vi "main_loop_calculation.vi"(0 "DAQ Data":waveform(dbl)[](array[waveform]), 1 "Offset Parameters":T1={"Separator \nTemperature"=0.0, "Separator Pressure"=0.0, "Lower Test Section\nTemperature"=0.0, "Lower Test Section\nPressure"=0.0, "Vapor Tank (Top) \nHeater"=0.0, "Liquid Tank (Bottom) \nHeater"=0.0, "Vapor Tank\nTemperature Offset"=0.0, "Vapor Tank\nPressure "=0.0, "Upper Test Section\nTemperature"=0.0, "Upper Test Section\nPressure"=0.0, "Vapor Inlet \nTemperature"=0.0, "Dev Section\nPressure"=0.0, "Liquid Tank\nTemperature"=0.0, "Liquid Tank\nPressure"=0.0, "Liquid Inlet\nTemperature "=0.0, "Liquid Inlet\nPressure"=0.0, "Atmospheric Pressure [Pa]"=101325.0}) -> (2 "Vapor Flow Data":T3, 3 "Liquid Flow Data":T2, 4 "Pressure/Temperature/Mixture Properties":T4)   [LabVIEW 2015]
panel:
  out "dt":dbl
  out "t0":timestamp
  out "Separator Temp. [C]":dbl
  out "Liquid Inlet T":dbl
  out "Vapor Inlet T Sat":dbl
  # "Saturation\nPressure [Pa]"
  # "Saturation\nTemperature [C]"
  # "Pressure [Pa]"
  # "Temperature [C]"
  # "Lower Test Section"
  # "Upper Test Section"
  # "Vapor Inlet\n(Dev Section)"
  # "Vapor Tank"
  # "Liquid Inlet"
  # "Separator"
  # "Liquid Tank"
  # "Streamwise(dP)"
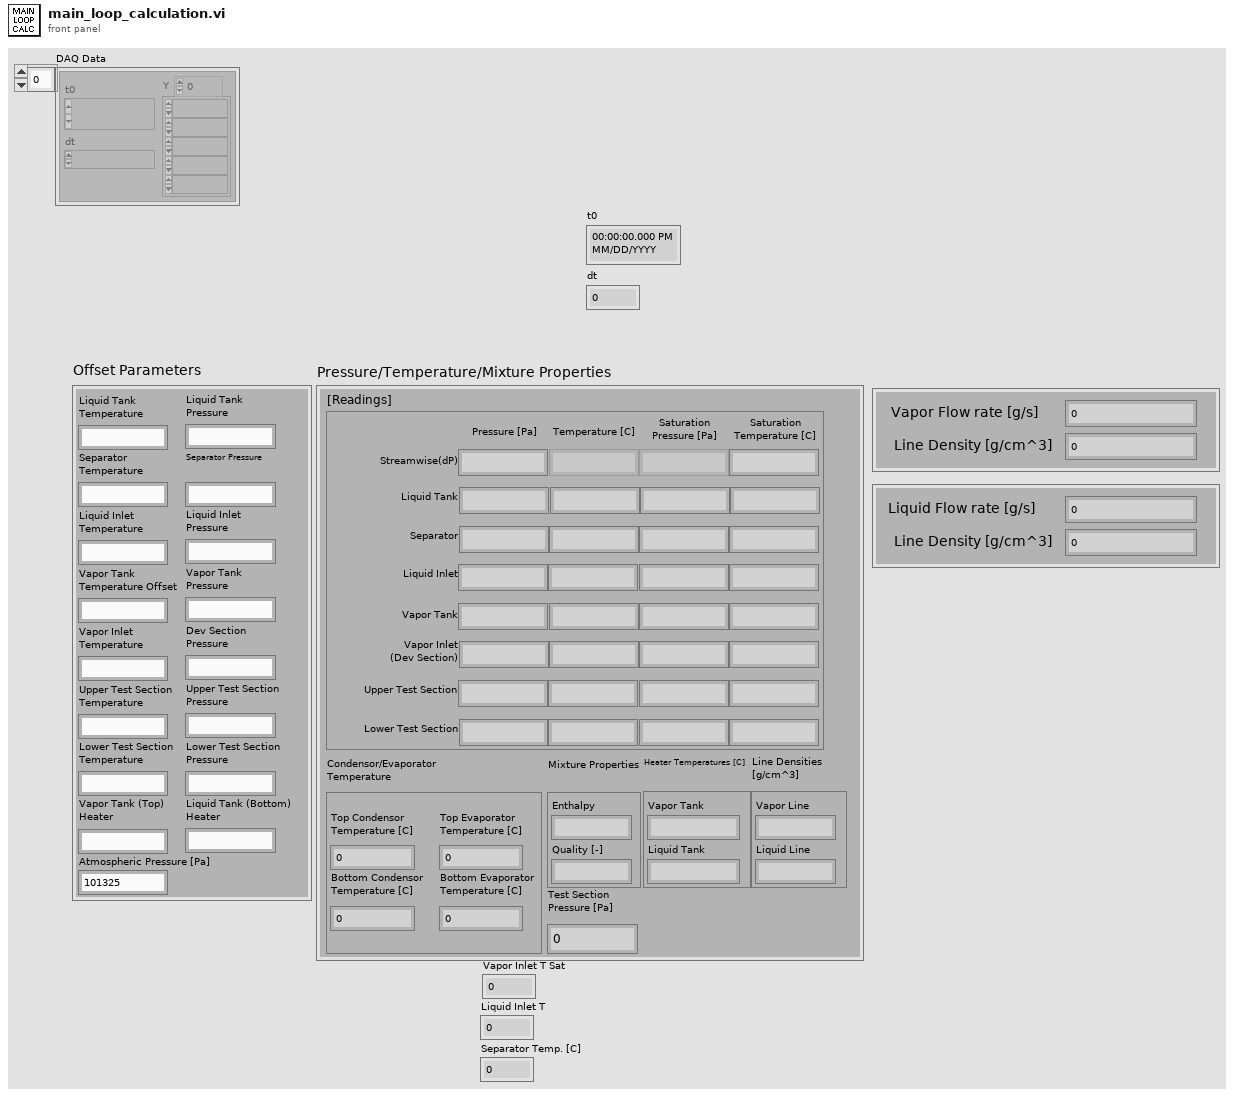
[diagram p1: front panel]
types:
  T1 = cluster{"Separator \nTemperature":dbl, "Separator Pressure":dbl, "Lower Test Section\nTemperature":dbl, "Lower Test Section\nPressure":dbl, "Vapor Tank (Top) \nHeater":dbl, "Liquid Tank (Bottom) \nHeater":dbl, "Vapor Tank\nTemperature Offset":dbl, "Vapor Tank\nPressure ":dbl, "Upper Test Section\nTemperature":dbl, "Upper Test Section\nPressure":dbl, "Vapor Inlet \nTemperature":dbl, "Dev Section\nPressure":dbl, "Liquid Tank\nTemperature":dbl, "Liquid Tank\nPressure":dbl, "Liquid Inlet\nTemperature ":dbl, "Liquid Inlet\nPressure":dbl, "Atmospheric Pressure [Pa]":dbl}
  T2 = cluster{"Liquid Flow rate [g/s]":dbl, "Line Density [g/cm^3]":dbl}
  T3 = cluster{"Vapor Flow rate [g/s]":dbl, "Line Density [g/cm^3]":dbl}
  T4 = cluster{"Line Densities\n[g/cm^3]":cluster{"Vapor Line":dbl, "Liquid Line":dbl}, "Mixture Properties":cluster{"Enthalpy":dbl, "Quality [-]":dbl}, "[Readings]":cluster{"Streamwise P":dbl, "Streamwise T":dbl, "Streamwise Sat P":dbl, "Streamwise Sat T":dbl, "Liquid Tank P":dbl, "Liquid Tank T":dbl, "Liquid Tank Sat P":dbl, "Liquid Tank Sat T":dbl, "Separator P":dbl, "Separator T":dbl, "Separator Sat P":dbl, "Separator Sat T":dbl, "Liquid Inlet P":dbl, "Liquid Inlet T":dbl, "Liquid Inlet Sat P":dbl, "Liquid Inlet Sat T":dbl, "Vapor Tank P":dbl, "Vapor Tank T":dbl, "Vapor Tank Sat P":dbl, "Vapor Tank Sat T":dbl, "Vapor Inlet P":dbl, "Vapor Inlet T":dbl, "Vapor Inlet Sat P":dbl, "Vapor Inlet Sat T":dbl, "Upper Test Section P":dbl, "Upper Test Section T":dbl, "Upper Test Section Sat P":dbl, "Upper Test Section Sat T":dbl, "Lower Test Section P":dbl, "Lower Test Section T":dbl, "Lower Test Section Sat P":dbl, "Lower Test Section Sat T":dbl}, "Condensor/Evaporator\nTemperature":cluster{"Bottom Evaporator\nTemperature [C]":dbl, "Bottom Condensor\nTemperature [C]":dbl, "Top Evaporator\nTemperature [C]":dbl, "Top Condensor\nTemperature [C]":dbl}, "Test Section \nPressure [Pa]":dbl, "Heater Temperatures [C]":cluster{"Vapor Tank":dbl, "Liquid Tank":dbl}}
  T5 = cluster{"[0]":dbl, "[1]":dbl, "[2]":dbl, "[3]":dbl}
  T6 = cluster{"mixture enthalpy":dbl, "Quality [-]":dbl}
  T7 = cluster{"array[0]":dbl, "array[1]":dbl, "array[2]":dbl, "array[3]":dbl, "array[4]":dbl, "array[5]":dbl, "array[6]":dbl, "array[7]":dbl, "array[8]":dbl, "array[9]":dbl, "array[10]":dbl, "array[11]":dbl, "array[12]":dbl, "array[13]":dbl, "array[14]":dbl, "array[15]":dbl, "array[16]":dbl, "array[17]":dbl, "array[18]":dbl, "array[19]":dbl, "array[20]":dbl, "array[21]":dbl, "array[22]":dbl, "array[23]":dbl, "array[24]":dbl, "array[25]":dbl, "array[26]":dbl, "array[27]":dbl, "array[28]":dbl, "array[29]":dbl, "array[30]":dbl, "array[31]":dbl}
  T8 = cluster{cluster{"[0]":dbl, "[1]":dbl}, cluster{"mixture enthalpy":dbl, "Quality [-]":dbl}, "Cluster":cluster{"array[0]":dbl, "array[1]":dbl, "array[2]":dbl, "array[3]":dbl, "array[4]":dbl, "array[5]":dbl, "array[6]":dbl, "array[7]":dbl, "array[8]":dbl, "array[9]":dbl, "array[10]":dbl, "array[11]":dbl, "array[12]":dbl, "array[13]":dbl, "array[14]":dbl, "array[15]":dbl, "array[16]":dbl, "array[17]":dbl, "array[18]":dbl, "array[19]":dbl, "array[20]":dbl, "array[21]":dbl, "array[22]":dbl, "array[23]":dbl, "array[24]":dbl, "array[25]":dbl, "array[26]":dbl, "array[27]":dbl, "array[28]":dbl, "array[29]":dbl, "array[30]":dbl, "array[31]":dbl}, cluster{"[0]":dbl, "[1]":dbl, "[2]":dbl, "[3]":dbl}, "Absolute Pressure [Pa]":dbl, cluster{"[0]":dbl, "[1]":dbl}}
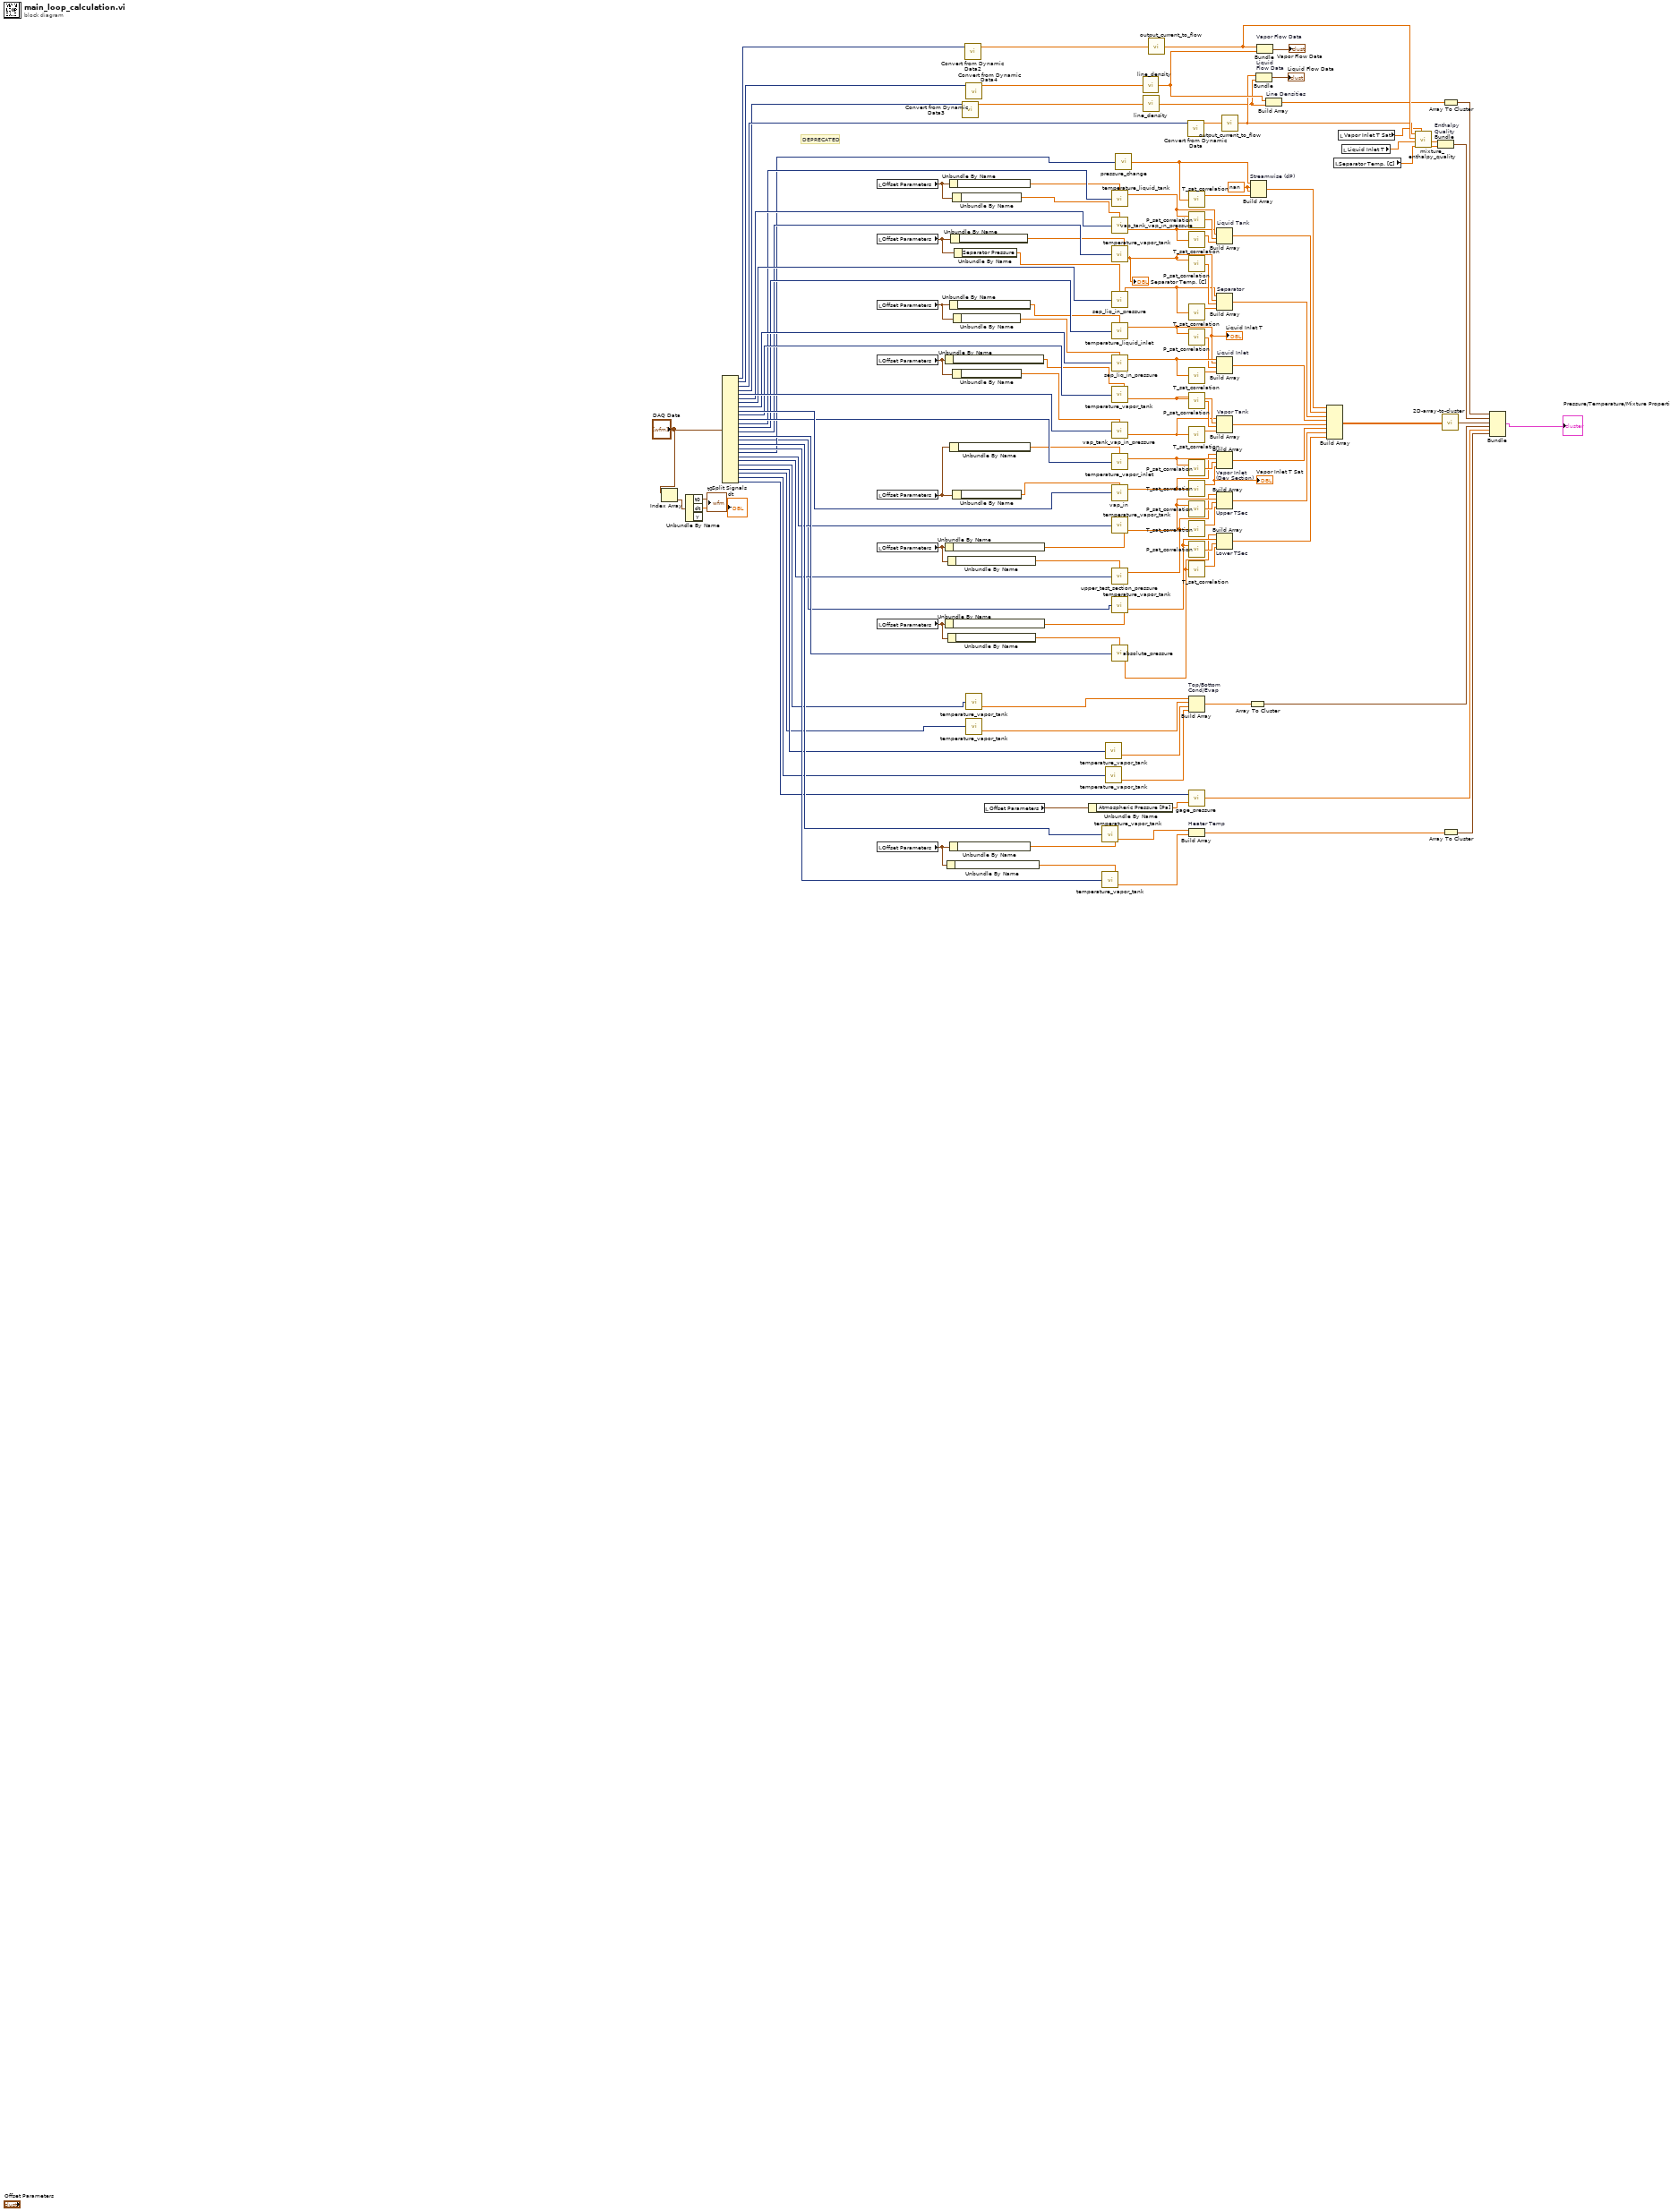
[diagram p0: block diagram]
diagram:
  w93 = nan
  # "DEPRECATED"
  n1 = Index Array(array="DAQ Data") -> (element=w3:waveform(dbl))  [unwired: 1 in]
  n2 = Unbundle By Name(w3) -> ("t0"=→"t0":timestamp, "dt"=→"dt":dbl)  [unwired: 1 out]
  n3 = Split Signals("DAQ Data") -> (w38:dynamicdata, w21:dynamicdata, w126:dynamicdata, w125:dynamicdata, w124:dynamicdata, w123:dynamicdata, w122:dynamicdata, w121:dynamicdata, w120:dynamicdata, w119:dynamicdata, w118:dynamicdata, w117:dynamicdata, w116:dynamicdata, w115:dynamicdata, w114:dynamicdata, w20:dynamicdata, w113:dynamicdata, w112:dynamicdata, w74:dynamicdata, w111:dynamicdata, w110:dynamicdata, w18:dynamicdata, w109:dynamicdata, w17:dynamicdata, w105:dynamicdata, w103:dynamicdata)  [unwired: 26 in]
  n4 = local read "Offset Parameters"() -> (w56:T1)
  n5 = local read "Offset Parameters"() -> (w52:T1)
  n6 = local read "Offset Parameters"() -> (w51:T1)
  n7 = local read "Offset Parameters"() -> (w58:T1)
  n8 = local read "Offset Parameters"() -> (w53:T1)
  n9 = local read "Offset Parameters"() -> (w54:T1)
  n10 = local read "Offset Parameters"() -> (w55:T1)
  n11 = local read "Offset Parameters"() -> (w57:T1)
  n12 = Unbundle By Name(w54) -> ("Upper Test Section\nTemperature"=w66:dbl)
  n13 = Unbundle By Name(w55) -> ("Lower Test Section\nTemperature"=w19:dbl)
  n14 = Unbundle By Name(w58) -> ("Vapor Tank\nTemperature Offset"=w68:dbl)
  n15 = Unbundle By Name(w57) -> ("Liquid Tank (Bottom) \nHeater"=w69:dbl)
  n16 = Unbundle By Name(w54) -> ("Upper Test Section\nPressure"=w65:dbl)
  n17 = Unbundle By Name(w55) -> ("Lower Test Section\nPressure"=w71:dbl)
  n18 = Unbundle By Name(w56) -> ("Liquid Tank\nTemperature"=w62:dbl)
  n19 = Unbundle By Name(w51) -> ("Liquid Inlet\nTemperature"=w60:dbl)
  n20 = Unbundle By Name(w57) -> ("Vapor Tank (Top) \nHeater"=w70:dbl)
  n21 = Unbundle By Name(w53) -> ("Vapor Inlet \nTemperature"=w64:dbl)
  n22 = Unbundle By Name(w52) -> ("Separator \nTemperature"=w73:dbl)
  n23 = Unbundle By Name(w56) -> ("Liquid Tank\nPressure"=w61:dbl)
  n24 = Unbundle By Name(w58) -> ("Vapor Tank\nPressure"=w67:dbl)
  n25 = Unbundle By Name(w53) -> ("Dev Section\nPressure"=w63:dbl)
  n26 = Unbundle By Name(w51) -> ("Liquid Inlet\nPressure"=w59:dbl)
  n27 = Unbundle By Name(w52) -> ("Separator Pressure"=w72:dbl)
  n28 = call "Convert from Dynamic Data3"("Dynamic Data Type"=w125) -> ("Array"=w23:dbl[])  [unwired: 3 in]
  n29 = call "Convert from Dynamic Data2"("Dynamic Data Type"=w38) -> ("Array"=w37:dbl[])  [unwired: 3 in]
  n30 = call "Convert from Dynamic Data4"("Dynamic Data Type"=w21) -> ("Array"=w22:dbl[])  [unwired: 3 in]
  n31 = call "temperature_vapor_tank.vi"("Temp. Voltage\n[V]"=w18) -> ("Offset Temp. [C]"=w108:dbl)  [unwired: 3 in]
  n32 = call "temperature_vapor_tank.vi"("Temp. Voltage\n[V]"=w17) -> ("Offset Temp. [C]"=w107:dbl)  [unwired: 3 in]
  n33 = local read "Offset Parameters"() -> (w42:T1)
  n34 = Unbundle By Name(w42) -> ("Atmospheric Pressure [Pa]"=w41:dbl)
  n35 = call "temperature_vapor_tank.vi"("Offset [C]"=w70, "Temp. Voltage\n[V]"=w113) -> ("Offset Temp. [C]"=w76:dbl)  [unwired: 2 in]
  n36 = call "temperature_vapor_tank.vi"("Offset [C]"=w69, "Temp. Voltage\n[V]"=w112) -> ("Offset Temp. [C]"=w75:dbl)  [unwired: 2 in]
  n37 = call "temperature_vapor_tank.vi"("Temp. Voltage\n[V]"=w109) -> ("Offset Temp. [C]"=w106:dbl)  [unwired: 3 in]
  n38 = call "temperature_vapor_tank.vi"("Temp. Voltage\n[V]"=w105) -> ("Offset Temp. [C]"=w104:dbl)  [unwired: 3 in]
  n39 = call "temperature_liquid_tank.vi"("Offset [C]"=w62, "Temp. Voltage\n[V]"=w117) -> ("Temp. [C]"=w102:dbl)  [unwired: 2 in, 1 out]
  n40 = call "vap_tank_vap_in_pressure.vi"("Offset [Pa]"=w61, "Abs. Pressure\nVoltage [V]"=w123) -> ("Offset Absolute Pressure [Pa]"=w88:dbl)  [unwired: 2 in, 1 out]
  n41 = call "temperature_vapor_tank.vi"("Offset [C]"=w73, "Temp. Voltage\n[V]"=w115) -> ("Offset Temp. [C]"=w35:dbl)  [unwired: 2 in]
  "Separator Temp. [C]" <- w35
  n42 = call "sep_liq_in_pressure.vi"("Offset [Pa]"=w72, "Abs. Pressure\nVoltage [V]"=w122) -> ("Absolute Pressure [Pa]"=w16:dbl)  [unwired: 2 in, 1 out]
  n43 = call "temperature_liquid_inlet.vi"("Offset [C]"=w60, "Temp. Voltage\n[V]"=w116) -> ("Temp. [C]"=w34:dbl)  [unwired: 2 in, 1 out]
  "Liquid Inlet T" <- w34
  n44 = call "sep_liq_in_pressure.vi"("Offset [Pa]"=w59, "Abs. Pressure\nVoltage [V]"=w121) -> ("Absolute Pressure [Pa]"=w85:dbl)  [unwired: 2 in, 1 out]
  n45 = call "temperature_vapor_tank.vi"("Offset [C]"=w68, "Temp. Voltage\n[V]"=w119) -> ("Offset Temp. [C]"=w92:dbl)  [unwired: 2 in]
  n46 = call "vap_tank_vap_in_pressure.vi"("Offset [Pa]"=w67, "Abs. Pressure\nVoltage [V]"=w124) -> ("Offset Absolute Pressure [Pa]"=w87:dbl)  [unwired: 2 in, 1 out]
  n47 = call "temperature_vapor_inlet.vi"("Offset [C]"=w64, "Temp. Voltage\n[V]"=w118) -> ("Temp. [C]"=w95:dbl)  [unwired: 2 in, 1 out]
  n48 = call "vap_in.vi"("Offset [Pa]"=w63, "Abs. Pressure\nVoltage [V]"=w120) -> ("Absolute Pressure [Pa]"=w24:dbl)  [unwired: 2 in, 1 out]
  n49 = call "temperature_vapor_tank.vi"("Offset [C]"=w66, "Temp. Voltage\n[V]"=w111) -> ("Offset Temp. [C]"=w78:dbl)  [unwired: 2 in]
  n50 = call "upper_test_section_pressure.vi"("Offset [Pa]"=w65, "Waveform Graph"=w110) -> ("Absolute Pressure [Pa]"=w77:dbl)  [unwired: 2 in, 1 out]
  n51 = call "temperature_vapor_tank.vi"("Offset [C]"=w19, "Temp. Voltage\n[V]"=w20) -> ("Offset Temp. [C]"=w91:dbl)  [unwired: 2 in]
  n52 = call "absolute_pressure.vi"("Offset [V]"=w71, "Abs. Pressure\nVoltage [V]"=w114) -> ("Offset Absolute Pressure [Pa]"=w86:dbl)  [unwired: 2 in, 1 out]
  n53 = call "pressure_change.vi"("Pressure Voltage (V)"=w74) -> ("Streamwise dP (kPa)"=w99:dbl)
  n54 = call "line_density.vi"("DensCurr"=w22) -> ("Line Density"=w29:dbl)
  n55 = call "line_density.vi"("DensCurr"=w23) -> ("Line Density"=w27:dbl)
  n56 = call "output_current_to_flow.vi"("Output Current"=w37) -> ("Flow rate"=w36:dbl)
  n57 = call "Convert from Dynamic Data"("Dynamic Data Type"=w126) -> ("Array"=w127:dbl[])  [unwired: 3 in]
  n58 = call "T_sat_correlation.vi"("P [Pa]"=w99) -> ("T Sat [C]"=w94:dbl)  [unwired: 1 out]
  n59 = call "P_sat_correlation.vi"("Temperature"=w102) -> ("P Sat"=w101:dbl)  [unwired: 1 in]
  n60 = call "T_sat_correlation.vi"("P [Pa]"=w88) -> ("T Sat [C]"=w100:dbl)  [unwired: 1 out]
  n61 = call "P_sat_correlation.vi"("Temperature"=w35) -> ("P Sat"=w82:dbl)  [unwired: 1 in]
  n62 = call "T_sat_correlation.vi"("P [Pa]"=w16) -> ("T Sat [C]"=w81:dbl)  [unwired: 1 out]
  n63 = call "P_sat_correlation.vi"("Temperature"=w34) -> ("P Sat"=w84:dbl)  [unwired: 1 in]
  n64 = call "T_sat_correlation.vi"("P [Pa]"=w85) -> ("T Sat [C]"=w83:dbl)  [unwired: 1 out]
  n65 = call "P_sat_correlation.vi"("Temperature"=w92) -> ("P Sat"=w97:dbl)  [unwired: 1 in]
  n66 = call "T_sat_correlation.vi"("P [Pa]"=w87) -> ("T Sat [C]"=w98:dbl)  [unwired: 1 out]
  n67 = call "P_sat_correlation.vi"("Temperature"=w95) -> ("P Sat"=w96:dbl)  [unwired: 1 in]
  n68 = call "T_sat_correlation.vi"("P [Pa]"=w24) -> ("T Sat [C]"=w9:dbl)  [unwired: 1 out]
  "Vapor Inlet T Sat" <- w9
  n69 = call "P_sat_correlation.vi"("Temperature"=w78) -> ("P Sat"=w80:dbl)  [unwired: 1 in]
  n70 = call "T_sat_correlation.vi"("P [Pa]"=w77) -> ("T Sat [C]"=w79:dbl)  [unwired: 1 out]
  n71 = call "P_sat_correlation.vi"("Temperature"=w91) -> ("P Sat"=w89:dbl)  [unwired: 1 in]
  n72 = call "T_sat_correlation.vi"("P [Pa]"=w86) -> ("T Sat [C]"=w90:dbl)  [unwired: 1 out]
  n73 = Build Array "Top/Bottom \nCond/Evap"(w108, w107, w106, w104) -> (w39:dbl[])
  n74 = call "gage_pressure.vi"("Atmospheric Pressure [Pa]"=w41, "Abs. Pressure\nVoltage [V]"=w103) -> ("Absolute Pressure [Pa]"=w11:dbl)
  n75 = Build Array "Heater Temp"(w76, w75) -> (w31:dbl[])
  n76 = Build Array "Liquid Tank"(w88, w102, w101, w100) -> (w45:dbl[])
  n77 = Build Array "Separator"(w16, w35, w82, w81) -> (w44:dbl[])
  n78 = Build Array "Liquid Inlet"(w85, w34, w84, w83) -> (w50:dbl[])
  n79 = Build Array "Vapor Tank"(w87, w92, w97, w98) -> (w49:dbl[])
  n80 = Build Array "Vapor Inlet\n(Dev Section)"(w24, w95, w96, w9) -> (w48:dbl[])
  n81 = Build Array "Upper TSec"(w77, w78, w80, w79) -> (w47:dbl[])
  n82 = Build Array "Lower TSec"(w86, w91, w89, w90) -> (w46:dbl[])
  n83 = call "output_current_to_flow.vi"("Output Current"=w127) -> ("Flow rate"=w28:dbl)
  n84 = Array To Cluster(array=w39) -> (cluster=w12:T5)
  n85 = Build Array "Streamwise (dP)"(w99, w93, w93, w94) -> (w43:dbl[])
  n86 = Bundle "Liquid\nFlow Data"("Flow rate"=w28, "Line Density"=w27) -> (→"Liquid Flow Data":cluster{"Flow rate":dbl, "Line Density":dbl})  [unwired: 1 in]
  n87 = Bundle "Vapor Flow Data"("Flow rate"=w36, "Line Density"=w29) -> (→"Vapor Flow Data":cluster{"Flow rate":dbl, "Line Density":dbl})  [unwired: 1 in]
  n88 = Build Array "Line Densities"(w29, w27) -> (w30:dbl[])
  n89 = Build Array(w43, w45, w44, w50, w49, w48, w47, w46) -> (w40:dbl[][])
  n90 = local read "Separator Temp. [C]"() -> (w8:dbl)
  n91 = local read "Vapor Inlet T Sat"() -> (w6:dbl)
  n92 = local read "Liquid Inlet T"() -> (w7:dbl)
  n93 = call "mixture_enthalpy_quality.vi"("Dev Section Pressure [Pa]"=w6, "Separator Temp [C]"=w8, "Liquid Inlet Temp [C]"=w7, "Vapor Flow Rate [g/s]"=w36, "Liquid Flow Rate [g/s]"=w28) -> ("Quality [-]"=w32:dbl, "mixture enthalpy"=w33:dbl)  [unwired: 2 out]
  n94 = Bundle "Enthalpy\nQuality"("mixture enthalpy"=w33, "Quality [-]"=w32) -> (w14:T6)  [unwired: 1 in]
  n95 = call "2D-array-to-cluster.vi"("2D Array"=w40) -> ("Cluster"=w15:T7)
  n96 = Array To Cluster(array=w30) -> (cluster=w13:cluster{"[0]":dbl, "[1]":dbl})
  n97 = Array To Cluster(array=w31) -> (cluster=w10:cluster{"[0]":dbl, "[1]":dbl})
  n98 = Bundle(w13, w14, "Cluster"=w15, w12, "Absolute Pressure [Pa]"=w11, w10) -> (→"Pressure/Temperature/Mixture Properties":T8)  [unwired: 1 in]
